vi "Initialize configuration property (object).vi"(6 "instance id":i32, 7 "vsObjectId":string, 8 "vsChIndex":i32, 9 "datatype":string, 10 "attribute name":string, 11 "class name":string) -> (3 "attribute configuration":T1)   [LabVIEW 2019, in "HLA Custom Device System Explorer.lvlib"]
uses:
  HLA Custom Device System Explorer.lvlib
  Shared/object_attribute_configuration.ctl
  Shared/HLA Custom Device Shared.lvlib
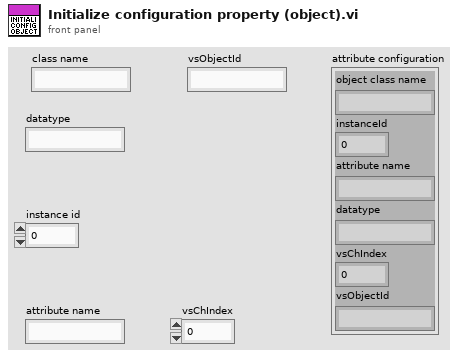
[diagram p1: front panel]
types:
  T1 = typedef "HLA Custom Device Shared.lvlib/object_attribute_configuration.ctl" = cluster{"object class name":string, "instanceId":i32, "attribute name":string, "datatype":string, "vsChIndex":i32, "vsObjectId":string}
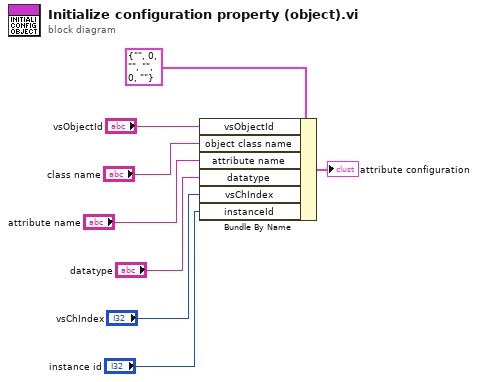
[diagram p0: block diagram]
diagram:
  n1 = Bundle By Name(cluster=T1 {"object class name"="", "instanceId"=0, "attribute name"="", "datatype"="", "vsChIndex"=0, "vsObjectId"=""}, "vsObjectId"="vsObjectId", "object class name"="class name", "attribute name"="attribute name", "datatype"="datatype", "vsChIndex"="vsChIndex", "instanceId"="instance id") -> (→"attribute configuration":T1)
